vi "Get Name.vi"(11 "iProcess Step Model in":refnum<class "iProcess Step Model.lvclass">) -> (1 "Name":string, 3 "iProcess Step Model out":refnum<class "iProcess Step Model.lvclass">)   [LabVIEW 2019, in "iProcess Step Model.lvclass"]
uses:
  <vilib>/gpm_packages/@cs/Car-wash/Source/iProcess Step Model/iProcess Step Model/iProcess Step Model.lvclass
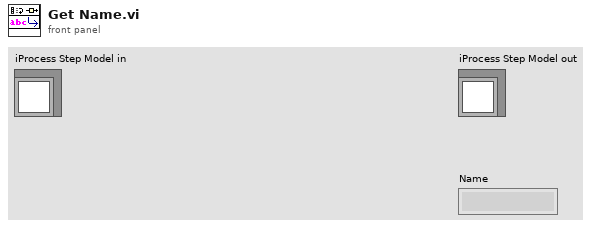
[diagram p1: front panel]
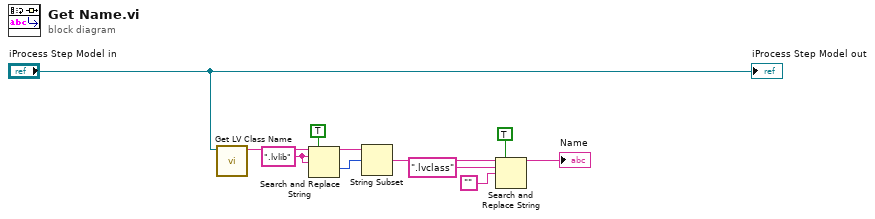
[diagram p0: block diagram]
diagram:
  w9 = ".lvlib" ("search string")
  n1 = call <vilib>:"Get LV Class Name.vi"("object"="iProcess Step Model in") -> ("class name"=w10:string)  [unwired: 9 in, 1 out]
  n2 = Search and Replace String(replace all?=TRUE ("replace all? (F)"), input string=w10, search string=w9, replace string=w9) -> (result string=w7:string, offset past replacement=w6:i32)  [unwired: 4 in, 2 out]
  n3 = String Subset(string=w7, offset (0)=w6) -> (substring=w5:string)  [unwired: 1 in]
  n4 = Search and Replace String(replace all?=TRUE ("replace all? (F)"), input string=w5, search string=".lvclass", replace string="") -> (result string=→"Name":string)  [unwired: 4 in, 3 out]
  "iProcess Step Model out" <- "iProcess Step Model in"
